vi "Close.vi"(8 "error in (no error)":errorcluster, 11 "VISA resource name":refnum<visa-resource-name>) -> (0 "error out":errorcluster)   [LabVIEW 2020, in "Datron D4xxx.lvlib"]
doc: "Performs an instrument error query before terminating the software connection to the instrument."
uses:
  Datron D4xxx.lvlib
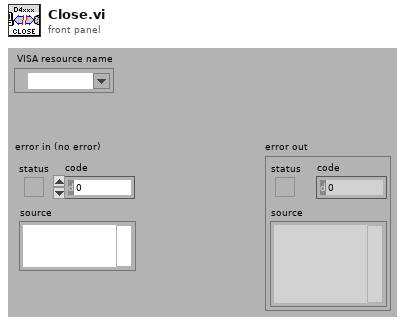
[diagram p1: front panel]
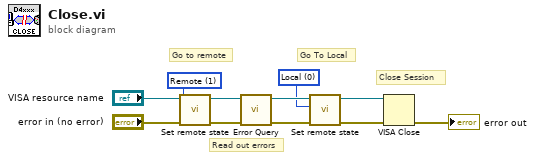
[diagram p0: block diagram]
diagram:
  w1 = u16 1 items=["Local", "Remote", "Default"] ("Remote state")
  w6 = u16 0 items=["Local", "Remote", "Default"] ("Remote state")
  # "Go to remote"
  # "Read out errors"
  # "Go To Local"
  # "Close Session"
  n1 = call "Set remote state.vi"("error in"="error in (no error)", "Remote state"=w1, "VISA resource name"="VISA resource name") -> ("error out"=w5:errorcluster, "VISA resource name out"=w4:refnum<visa-resource-name>)  [unwired: 7 in]
  n2 = call "Error Query.vi"("error in (no error)"=w5, "VISA resource name"=w4) -> ("error out"=w10:errorcluster, "VISA resource name out"=w9:refnum<visa-resource-name>)  [unwired: 6 in, 2 out]
  n3 = call "Set remote state.vi"("error in"=w10, "Remote state"=w6, "VISA resource name"=w9) -> ("error out"=w8:errorcluster, "VISA resource name out"=w7:refnum<visa-resource-name>)  [unwired: 7 in]
  n4 = VISA Close(VISA resource name=w7, error in (no error)=w8) -> (error out=→"error out":errorcluster)
